vi "battlesonCH#1.vi"   [LabVIEW 2014, in "Battleson_Robot_12-2-16.lvrbt"]
uses:
  Battleson_Robot_12-2-16.lvrbt
  <vilib>/NXT/Block Support/NXT_InputPort.ctl
  <vilib>/NXT/Block Support/NXT_OutputPort.ctl
  <vilib>/NXT/NXTIO Xnodes/NXTIONodeSubVIs/NXTMoveMotors.vi
  <vilib>/NXT/Dual Mode Library/Waits/Wait_Num.vi
  <vilib>/NXT/NXTIO Xnodes/NXTIONodeSubVIs/LEGOStopAllMotors.vi
  <vilib>/NXT/NXTIO Xnodes/AddressXNode/NXTIOAddress.xnode
  <vilib>/NXT/NXTIO Xnodes/NXTIOXNode/NXTIO.xnode
  <vilib>/NXT/Subs/LVHSConnector.ctl
  <vilib>/NXT/LegoClasses/BrickReference/BrickReference.lvclass
types:
  T1 = typedef "NXT_OutputPort.ctl" = u8
  T2 = typedef "NXT_InputPort.ctl" = u32
  T3 = typedef "LVHSConnector.ctl" = refnum<class "BrickReference.lvclass">
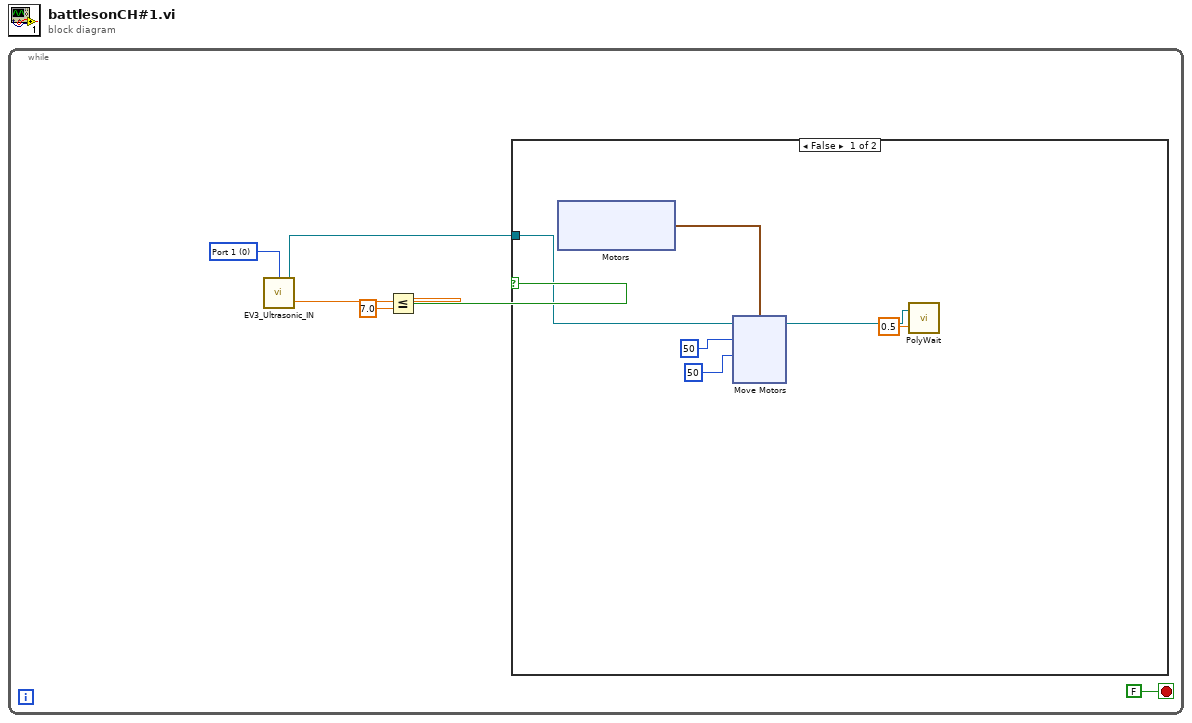
[diagram p0: block diagram]
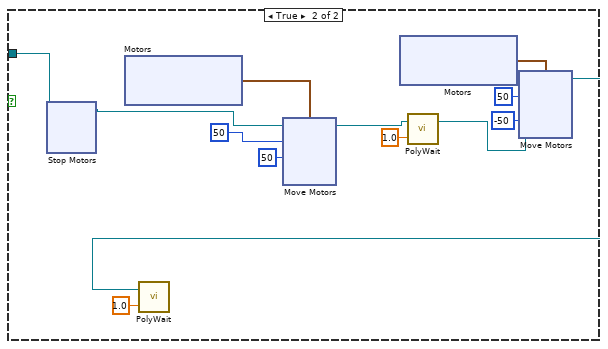
[diagram p2: hidden frame]
diagram:
  n1 = while {
    stop <- FALSE stop-if-true
    w1 = T2 0 items=["Port 1", "Port 2", "Port 3", "Port 4"] ("Port (Port 1)")
    n2 = call <vilib>:"EV3_Ultrasonic_IN.vi"("Port (Port 1)"=w1) -> ("Inches"=w3:sgl, "NXT/EV3"=w4:T3)  [unwired: 2 in]
    n3 = Less Or Equal?(x=w3, y=sgl 7.0) -> (x <= y?=w5:bool)
    n4 = case shown="False" w5 {
      tunnel: w4 -> [w11 w25]
      frame False {
        n5 = xnode "Motors"() -> ("Motor"=w12:cluster{"Port":T1, "Port":T1})
        n6 = xnode "Move Motors"("Power/Speed 2"=i8 50, "Power/Speed 1"=i8 50, "Motors"=w12, "NXT/EV3"=w11) -> ("NXT/EV3"=w10:T3)
        n7 = call-poly <vilib>:"PolyWait.vi"("Time (1 sec)"=sgl 0.5, "NXT/EV3"=w10) -> ()  [unwired: 2 in, 1 out]
      }
      frame True {
        n8 = xnode "Stop Motors"("NXT/EV3"=w25) -> ("NXT/EV3"=w24:T3)  [unwired: 1 in]
        n9 = xnode "Motors"() -> ("Motor"=w34:cluster{"Port":T1, "Port":T1})
        n10 = xnode "Move Motors"("Power/Speed 2"=i8 50, "Power/Speed 1"=i8 50, "Motors"=w34, "NXT/EV3"=w24) -> ("NXT/EV3"=w32:T3)
        n11 = xnode "Motors"() -> ("Motor"=w30:cluster{"Port":T1, "Port":T1})
        n12 = call-poly <vilib>:"PolyWait.vi"("Time (1 sec)"=sgl 1.0, "NXT/EV3"=w32) -> ("NXT/EV3"=w23:T3)  [unwired: 2 in]
        n13 = xnode "Move Motors"("Power/Speed 2"=i8 -50, "Power/Speed 1"=i8 50, "Motors"=w30, "NXT/EV3"=w23) -> ("NXT/EV3"=w27:T3)
        n14 = call-poly <vilib>:"PolyWait.vi"("Time (1 sec)"=sgl 1.0, "NXT/EV3"=w27) -> ()  [unwired: 2 in, 1 out]
      }
    }
  }
